vi "Read Motor Command.vi"(8 "error in (no error)":errorcluster, 11 "MCB Command in":refnum<class "MCB Command.lvclass">) -> (0 "error out":errorcluster, 1 "Motor Command":i16, 2 "Motor":T1, 3 "MCB Command out":refnum<class "MCB Command.lvclass">)   [LabVIEW 2015, in "RDS Child Messages.lvlib" / "MCB Command.lvclass"]
uses:
  MCB Command.lvclass
  MCB Channel.ctl
  MCB Command.lvclass/MCB Command.ctl
  RDS Child Messages.lvlib
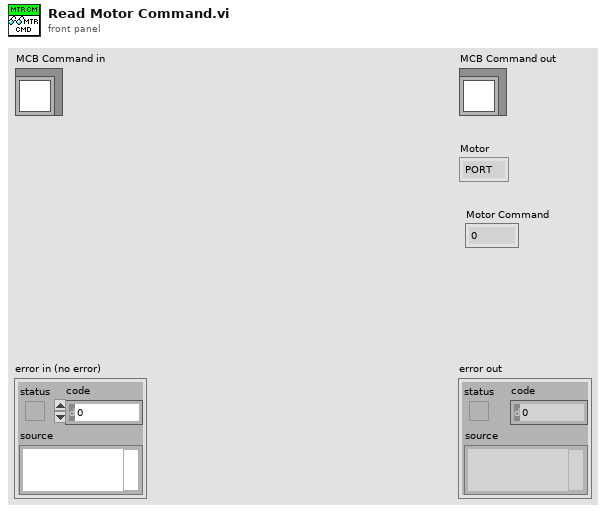
[diagram p1: front panel]
types:
  T1 = typedef "RDS Child Messages.lvlib/MCB Channel.ctl" = enum16{"PORT", "STBD"}
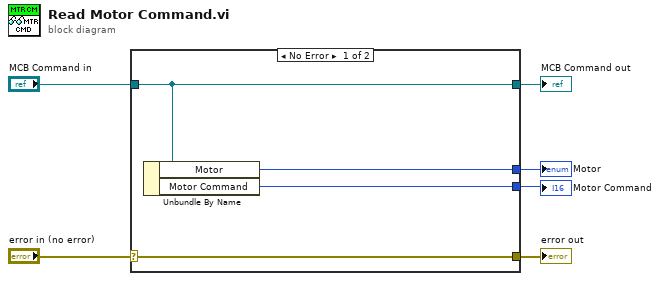
[diagram p0: block diagram]
diagram:
  n1 = case shown="No Error" "error in (no error)" {
    selector: "error in (no error)" -> [w10 w11]
    tunnel: [w10 w11] -> w5
    tunnel: [w9 w12] -> w3
    tunnel: "MCB Command in" -> [w9 w12]
    tunnel: [w8 _] -> w2
    tunnel: [w7 _] -> w1
    frame No Error {
      n2 = Unbundle By Name(w9) -> ("Motor"=w8:T1, "Motor Command"=w7:i16)
    }
    frame Error {
    }
  }
  "error out" <- w5
  "MCB Command out" <- w3
  "Motor" <- w2
  "Motor Command" <- w1
